vi "MCP4725_with_GraphforLoop.vi"() -> ()   [LabVIEW 2017]
uses:
  <vilib>/MakerHub/LINX/Public/Peripherals/Analog/Analog Read 1 Chan.vi
  <vilib>/MakerHub/LINX/Private/Local IO/LinxI2cWrite.vi
  <vilib>/MakerHub/LINX/Public/Utilities/Check Channel.vi
  <vilib>/MakerHub/LINX/Public/Peripherals/Analog/Analog Read N Chans.vi
  <vilib>/MakerHub/LINX/Private/Local IO/LinxAnalogRead.vi
  <vilib>/MakerHub/LINX/Public/Utilities/Open Serial.vi
  <vilib>/MakerHub/LINX/Private/Utilties/Generate Error.vi
  <vilib>/MakerHub/LINX/LMH-LINX.lvlib
panel:
  out "output array":dbl[](array[numeric])
  out "XY Graph":cluster{dbl[], dbl[]}(graph)
  in  "Select Analog Channel\nto be Read":u8
  out "Voltage on Analog Channel;":dbl(knob) scale=0.0..5.0
  out "Current Value written to \nDAC  input":u16
  out "Device Name":string
  out "Error Out":errorcluster
  in  "Data Collection\nTime  Interval (ms)":u32
  in  "Arduino \nSerial Port":refnum<visa-resource-name>="N/A"
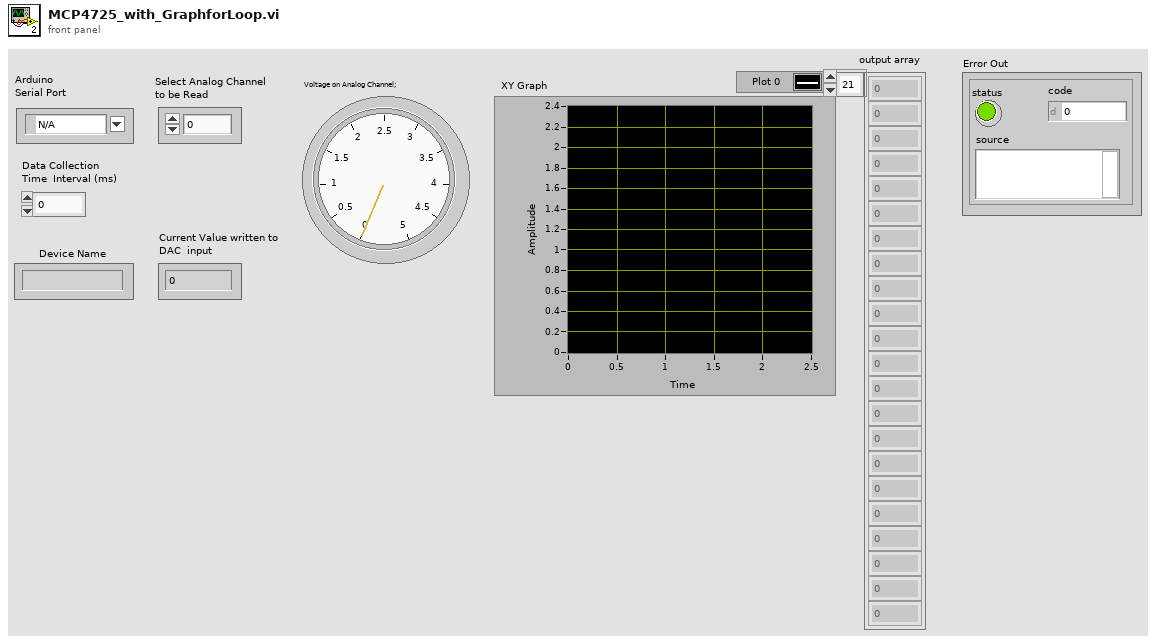
[diagram p1: front panel]
types:
  T1 = typedef "LMH-LINX.lvlib/LINX Ref.ctl" = cluster{"IO":T2, "Interface":T3, "LINX Device Config":T4}
  T2 = typedef "LMH-LINX.lvlib/Platform.ctl" = enum16{"Remote", "Local"}
  T3 = typedef "LMH-LINX.lvlib/Interface.ctl" = enum16{"Serial", "TCP"}
  T4 = typedef "LMH-LINX.lvlib/Device.lvlib/LINX Device Config.ctl" = cluster{"Interface":T3, "COM Port":refnum<visa-resource-name>, "TCP Configuration":T5, "Device Family":u8, "Device ID":u8, "Device Name":string, "TCP Ref":refnum<k5>, "Channels":T6}
  T5 = typedef "LMH-LINX.lvlib/Device.lvlib/TCP Config.ctl" = cluster{"IP Address":string, "Port":u16}
  T6 = typedef "LMH-LINX.lvlib/Channels.ctl" = cluster{"DI":u8[], "DO":u8[], "AI":u8[], "AO":u8[], "PWM":u8[], "QE":u8[], "UART":u8[], "I2C 2":u8[], "SPI":u8[], "CAN":u8[], "Servo":u8[], "AI Ref (V)":dbl, "AI Resolution (Bits)":u8, "AO Ref (V)":dbl, "AO Resolution (Bits)":u8}
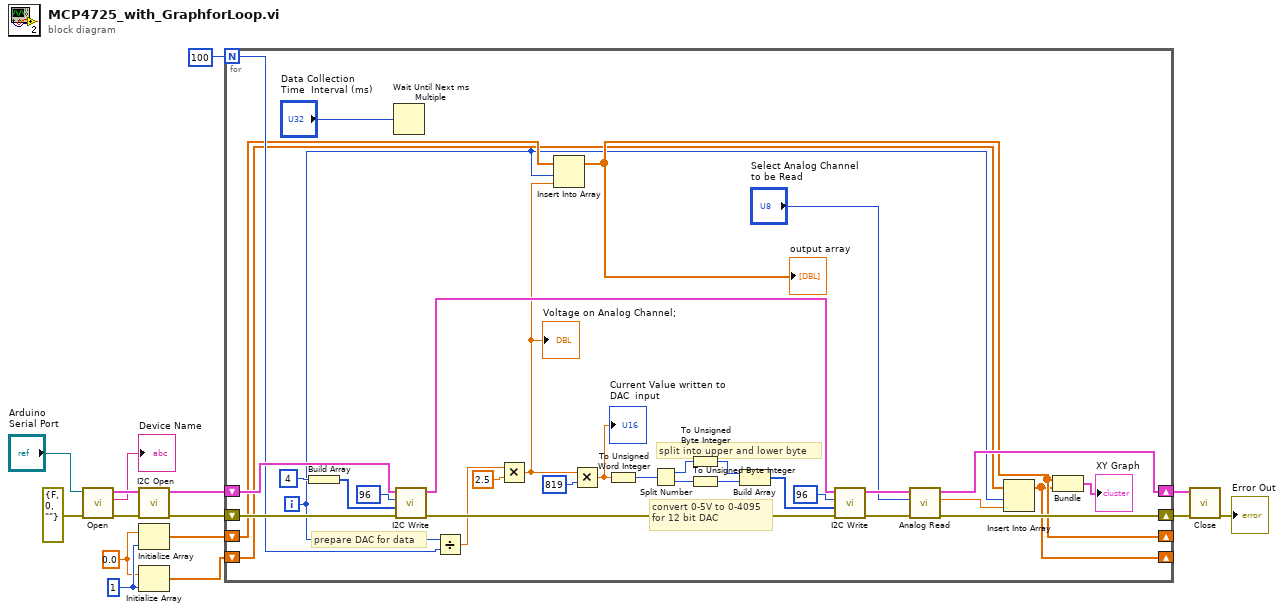
[diagram p0: block diagram]
diagram:
  w4 = 0.0 ("element")
  w5 = 1 ("dimension size")
  n1 = call-poly <vilib>:"Open.vi"("Error In"=errorcluster {"status"=FALSE, "code"=0, "source"=""}, "Serial Port"="Arduino \nSerial Port") -> ("Error Out"=w13:errorcluster, "Device Name"=→"Device Name":string, "LINX Resource"=w14:T1)  [unwired: 7 in]
  n2 = call <vilib>:"I2C Open.vi"("Error In"=w13, "LINX Resource"=w14) -> ("Error Out"=w10:errorcluster, "LINX Resource"=w11:T1)  [unwired: 8 in]
  n3 = Initialize Array(w4, w5) -> (w3:dbl[])
  n4 = Initialize Array(w4, w5) -> (w2:dbl[])
  n5 = for {
    N: 100 -> [w25]
    shift-right: [w30] -> w7
    shift-left: w11 -> [w48]
    shift-right: [w28] -> w6
    shift-left: w10 -> [w47]
    shift-right: [w20] -> _
    shift-left: w3 -> [w21]
    shift-right: [w18] -> _
    shift-left: w2 -> [w19]
    i -> [w16]
    # "prepare DAC for data"
    # "convert 0-5V to 0-4095\nfor 12 bit DAC"
    # "split into upper and lower byte"
    n6 = Build Array(u8 4) -> (w32:u8[])
    n7 = Wait Until Next ms Multiple(millisecond multiple="Data Collection\nTime  Interval (ms)") -> ()  [unwired: 1 out]
    n8 = call <vilib>:"I2C Write.vi"("Error In"=w47, "Data"=w32, "I2C Slave Address (0)"=u8 96, "LINX Resource"=w48) -> ("Error Out"=w36:errorcluster, "LINX Resource"=w35:T1)  [unwired: 6 in]
    n9 = Divide(x=w16, y=w25) -> (x/y=w24:dbl)
    n10 = Multiply(x=w24, y=2.5) -> (x*y=w23:dbl)
    "Voltage on Analog Channel;" <- w23
    n11 = Insert Into Array(array=w21, index=w16, new element=w23) -> (w20:dbl[])
    "output array" <- w20
    n12 = Multiply(x=w23, y=u32 819) -> (x*y=w34:dbl)
    "Current Value written to \nDAC  input" <- w34
    n13 = To Unsigned Word Integer(number=w34) -> (unsigned 16bit integer=w39:u16)
    n14 = Split Number(x=w39) -> (hi(x)=w40:u8, lo(x)=w45:u8)
    n15 = To Unsigned Byte Integer(number=w40) -> (unsigned 8bit integer=w43:u8)
    n16 = To Unsigned Byte Integer(number=w45) -> (unsigned 8bit integer=w42:u8)
    n17 = Build Array(w43, w42) -> (w41:u8[])
    n18 = call <vilib>:"I2C Write.vi"("Error In"=w36, "Data"=w41, "I2C Slave Address (0)"=u8 96, "LINX Resource"=w35) -> ("Error Out"=w29:errorcluster, "LINX Resource"=w31:T1)  [unwired: 6 in]
    n19 = call-poly <vilib>:"Analog Read.vi"("Error In"=w29, "Analog Channel"="Select Analog Channel\nto be Read", "LINX Resource"=w31) -> ("Error Out"=w28:errorcluster, "Voltage"=w17:dbl, "LINX Resource"=w30:T1)  [unwired: 5 in, 1 out]
    n20 = Insert Into Array(array=w19, index=w16, new element=w17) -> (w18:dbl[])
    n21 = Bundle(w20, w18) -> (→"XY Graph":cluster{dbl[], dbl[]})  [unwired: 1 in]
  }
  n22 = call <vilib>:"Close.vi"("Error In"=w6, "LINX Resource"=w7) -> ("Error Out"=→"Error Out":errorcluster)  [unwired: 9 in]
